vi "BoolDec.vi"(0 "Bit0":bool, 1 "Bit1":bool, 2 "Bit2":bool, 3 "Bit3":bool) -> (8 "Out":i8)   [LabVIEW 2018]
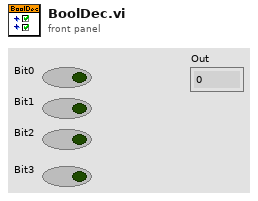
[diagram p1: front panel]
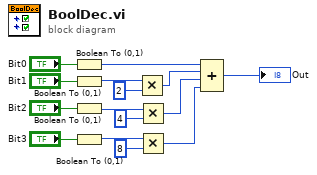
[diagram p0: block diagram]
diagram:
  n1 = Boolean To (0,1)(Boolean="Bit0") -> (0, 1=w13:i16)
  n2 = Boolean To (0,1)(Boolean="Bit1") -> (0, 1=w12:i16)
  n3 = Boolean To (0,1)(Boolean="Bit2") -> (0, 1=w4:i16)
  n4 = Boolean To (0,1)(Boolean="Bit3") -> (0, 1=w3:i16)
  n5 = Multiply(x=w12, y=i8 2) -> (x*y=w14:i16)
  n6 = Multiply(x=w4, y=i8 4) -> (x*y=w2:i16)
  n7 = Multiply(x=w3, y=i8 8) -> (x*y=w1:i16)
  n8 = Compound Arithmetic op=ADD(w13, w14, w2, w1) -> (→"Out":i16)
